vi "Xbox.vi"() -> ()   [LabVIEW 2014]
panel:
  in  "hi":bool
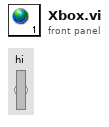
[diagram p1: front panel]
diagram:
